vi "Drive Straight.vi"(2 "Rate L":dbl, 3 "Rate R":dbl, 4 "Speed":dbl(slide) scale=0.0..0.75) -> (0 "Y Out":dbl, 1 "X Out":dbl)   [LabVIEW 2015]
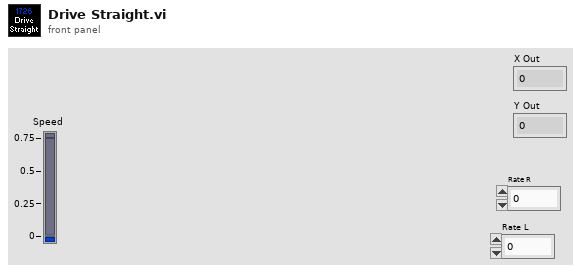
[diagram p1: front panel]
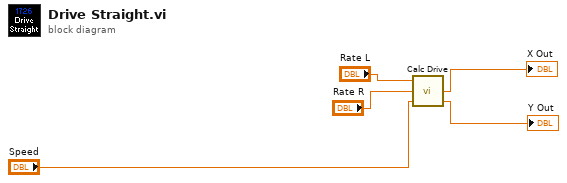
[diagram p0: block diagram]
diagram:
  n1 = call "Calc Drive.vi"("Target Speed"="Speed", "Rate Right"="Rate R", "Rate Left"="Rate L") -> ("Y Out"=→"Y Out":dbl, "X Out"=→"X Out":dbl)  [unwired: 1 in]
